vi "Synapse Initialize - Callback.vi"(4 "user event out":refnum<user-event>, 5 "Event Data":cluster{"status":i32, "eventInfo":refnum<k7>}, 6 "Control Ref":refnum<k7>, 7 "Event Common Data":T1) -> ()   [LabVIEW 2023]
doc: "This VI gets called when the CCD is initialized; it signals that it has been called by generating a (boolean) user event, which normally is used to trigger an event structure in the calling VI. (This allows the calling VI to pause until the event is received.)"
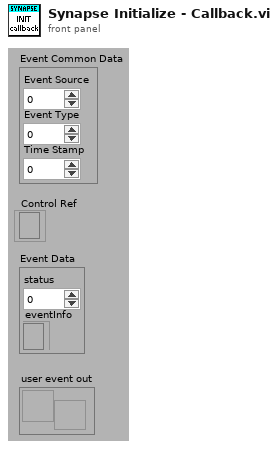
[diagram p1: front panel]
types:
  T1 = cluster{"Event Source":i32, "Event Type":u32, "Time Stamp":u32}
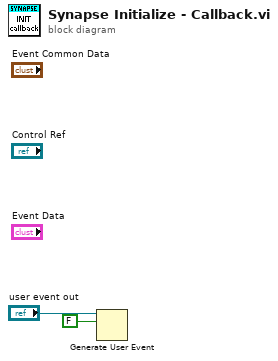
[diagram p0: block diagram]
diagram:
  n1 = Generate User Event(user event="user event out", event data cluster=FALSE ("event data")) -> ()  [unwired: 2 in, 2 out]
